vi "Snap to +-180.vi"(1 "Slide":dbl(slide) scale=-1000.0..1000.0) -> (0 "Slide 2":dbl(slide) scale=-1000.0..1000.0)   [LabVIEW 2019]
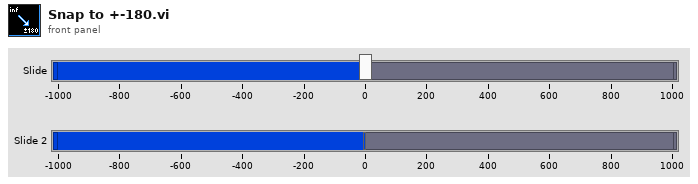
[diagram p1: front panel]
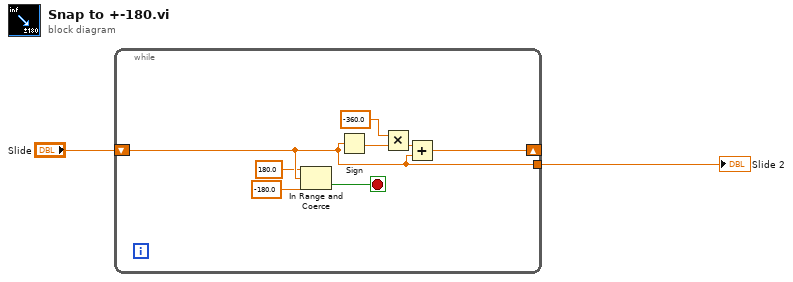
[diagram p0: block diagram]
diagram:
  n1 = while {
    shift-right: [w6] -> _
    shift-left: "Slide" -> [w5]
    tunnel: [w5] -> w1
    stop <- w10 stop-if-true
    n2 = In Range and Coerce(upper limit=180.0, x=w5, lower limit=-180.0) -> (In Range?=w10:bool)  [unwired: 1 out]
    n3 = Sign(1:w5) -> (0:w9:dbl)
    n4 = Multiply(x=-360.0, y=w9) -> (x*y=w7:dbl)
    n5 = Add(x=w7, y=w5) -> (x+y=w6:dbl)
  }
  "Slide 2" <- w1
